vi "ReadEncDrive.vi"(5 "Teleop Local Data":T1 {"Vision"."Theta_Y" format="%.1f"; "Vision"."Theta_X" format="%.1f"; "Potentio" format="%.1f"; "Drive_Enc_R" format="%.1f"; "Drive_Enc_L" format="%.1f"; "Gyro_Angle" format="%.1f"; "Encoder_Lift" format="%.1f"; "Motor_Lift" format="%.3f"; "Motor_Intake" format="%.3f"; "Drive_Twist" format="%.3f"; "Drive_Forward" format="%.3f"}, 9 "error in":errorcluster) -> (6 "Teleop Local Data Out":T1 {"Vision"."Theta_Y" format="%.1f"; "Vision"."Theta_X" format="%.1f"; "Potentio" format="%.1f"; "Drive_Enc_R" format="%.1f"; "Drive_Enc_L" format="%.1f"; "Gyro_Angle" format="%.1f"; "Encoder_Lift" format="%.1f"; "Motor_Lift" format="%.3f"; "Motor_Intake" format="%.3f"; "Drive_Twist" format="%.3f"; "Drive_Forward" format="%.3f"}, 10 "error out":errorcluster)   [LabVIEW 2018]
uses:
  Typedefs/typedef_cluster_TeleOp_Local_Data.ctl
  Typedefs/typedef_cluster_Joystick.ctl
  Typedefs/typedef_cluster_Vision.ctl
  Typedefs/typedef_enum_refnums.ctl
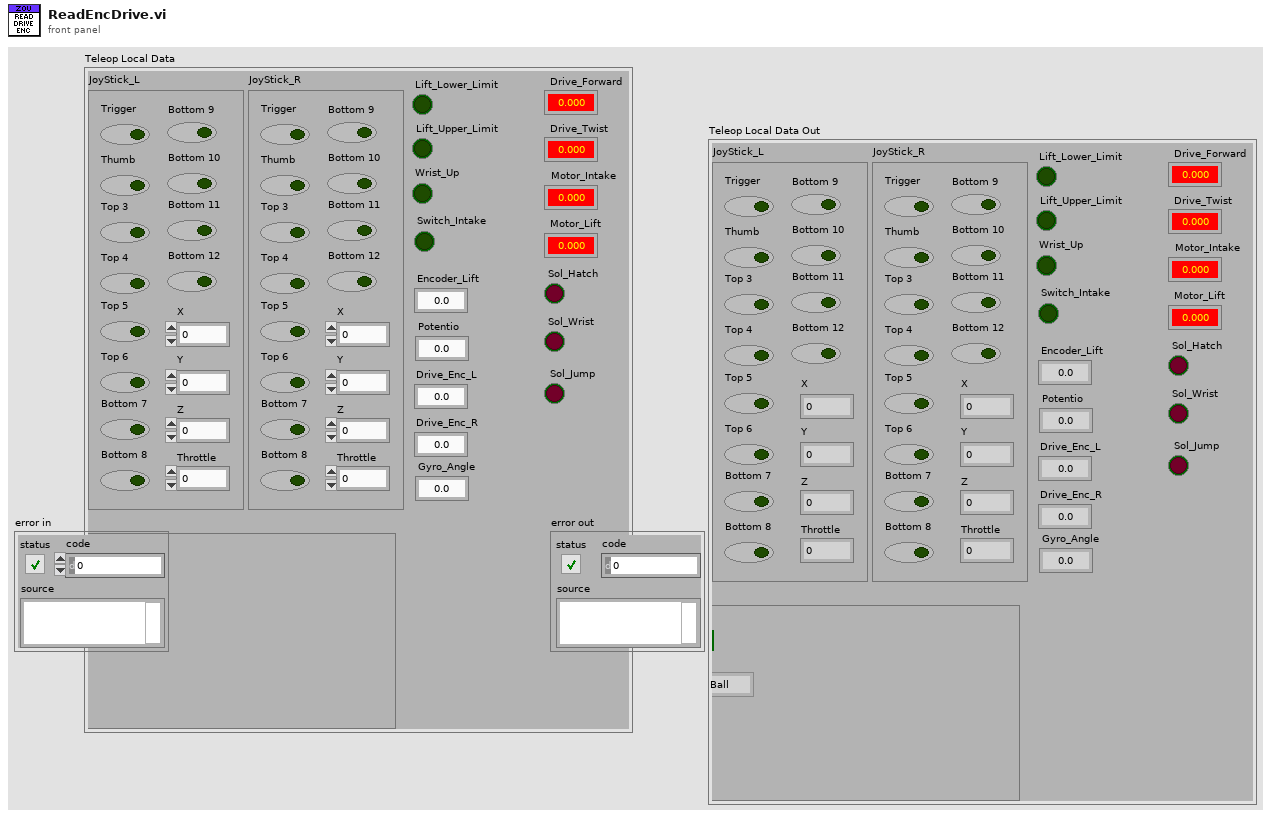
[diagram p1: front panel]
types:
  T1 = typedef "typedef_cluster_TeleOp_Local_Data.ctl" = cluster{"Lift_Lower_Limit":bool, "Wrist_Up":bool, "Switch_Intake":bool, "Encoder_Lift":dbl, "Sol_Wrist":bool, "Motor_Intake":dbl, "Motor_Lift":dbl, "Drive_Forward":dbl, "Drive_Twist":dbl, "Sol_Hatch":bool, "Gyro_Angle":dbl, "Drive_Enc_L":dbl, "Drive_Enc_R":dbl, "JoyStick_L":T2, "JoyStick_R":T2, "Potentio":dbl, "Vision":T3, "Lift_Upper_Limit":bool, "Sol_Jump":bool}
  T2 = typedef "typedef_cluster_Joystick.ctl" = cluster{"X":dbl, "Y":dbl, "Z":dbl, "Throttle":dbl, "Trigger":bool, "Thumb":bool, "Top 3":bool, "Top 4":bool, "Top 5":bool, "Top 6":bool, "Bottom 7":bool, "Bottom 8":bool, "Bottom 9":bool, "Bottom 10":bool, "Bottom 11":bool, "Bottom 12":bool}
  T3 = typedef "typedef_cluster_Vision.ctl" = cluster{"Theta_X":dbl, "Theta_Y":dbl, "Has_Target":bool, "Seek_Ball":bool, "Pipeline":enum16{"Ball", "Dual_Target", "Single_Target"}}
  T4 = typedef "typedef_enum_refnums.ctl" = enum16{"Joy_L", "Joy_R", "Drive_Motors", "Intake_Motor", "Wrist_Solenoid", "Hatch_Solenoid", "Compressor", "Lift_Motor", "Lift_Motor_2", "Gyro", "Drive_Enc_L", "Drive_Enc_R", "Lift_Lower_Limit", "Lift_Upper_Limit", "Ball_Switch", "Jump_Solenoid"}
  T5 = typedef "WPI_EncoderDevRef.ctl" = cluster{"DevStatus":errorcluster, "EncoderIndex":T6, "CounterIndex":T7, "DistancePerCount":dbl, "Decoding Type":T8}
  T6 = typedef "FPGA_EncoderIdx.ctl" = enum8{"Enc 0", "Enc 1", "Enc 2", "Enc 3", "Enc 4", "Enc 5", "Enc 6", "Enc 7", "Invalid"}
  T7 = typedef "FPGA_CounterCtrSystemIndex.ctl" = enum8{"Ctr 0", "Ctr 1", "Ctr 2", "Ctr 3", "Ctr 4", "Ctr 5", "Ctr 6", "Ctr 7", "Invalid"}
  T8 = typedef "WPI_EncoderType.ctl" = enum16{"1x", "2x", "4x"}
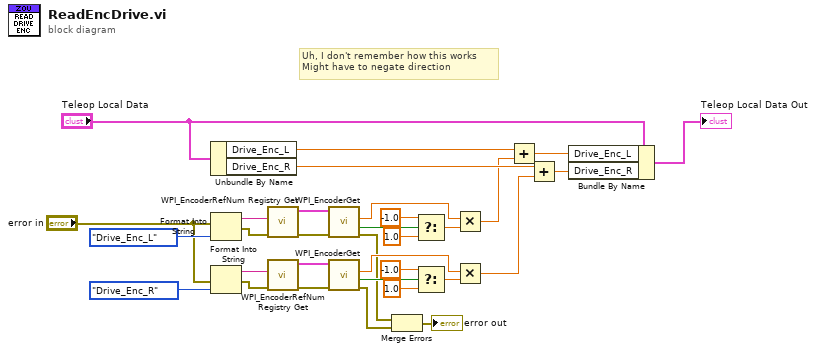
[diagram p0: block diagram]
diagram:
  # "Uh, I don't remember how this works\nMight have to negate direction"
  n1 = Unbundle By Name("Teleop Local Data") -> ("Drive_Enc_L"=w11:dbl, "Drive_Enc_R"=w12:dbl)
  n2 = Format Into String(error in="error in", typedef_enum_refnums."Drive_Enc_L" ("Enum")) -> (resulting string=w30:string, error out=w7:errorcluster)  [unwired: 2 in]
  n3 = Format Into String(error in="error in", typedef_enum_refnums."Drive_Enc_R" ("Enum")) -> (resulting string=w29:string, error out=w5:errorcluster)  [unwired: 2 in]
  n4 = call <vilib>:"WPI_EncoderRefNum Registry Get.vi"("error in (no error)"=w7, "refnum name"=w30) -> ("error out"=w6:errorcluster, "EncoderDevRef"=w27:T5)  [unwired: 8 in]
  n5 = call <vilib>:"WPI_EncoderRefNum Registry Get.vi"("error in (no error)"=w5, "refnum name"=w29) -> ("error out"=w4:errorcluster, "EncoderDevRef"=w28:T5)  [unwired: 8 in]
  n6 = call <vilib>:"WPI_EncoderGet.vi"("error in (no error)"=w6, "EncoderDevRef"=w27) -> ("error out"=w3:errorcluster, "Direction"=w22:bool, "Distance"=w20:dbl)  [unwired: 4 in, 3 out]
  n7 = call <vilib>:"WPI_EncoderGet.vi"("error in (no error)"=w4, "EncoderDevRef"=w28) -> ("error out"=w2:errorcluster, "Direction"=w16:bool, "Distance"=w15:dbl)  [unwired: 4 in, 3 out]
  n8 = Merge Errors(w3, w2) -> (→"error out":errorcluster)
  n9 = Select(t=-1.0, s=w22, f=1.0) -> (s? t:f=w21:dbl)
  n10 = Select(t=-1.0, s=w16, f=1.0) -> (s? t:f=w19:dbl)
  n11 = Multiply(x=w20, y=w21) -> (x*y=w10:dbl)
  n12 = Multiply(x=w15, y=w19) -> (x*y=w9:dbl)
  n13 = Add(x=w11, y=w10) -> (x+y=w14:dbl)
  n14 = Add(x=w12, y=w9) -> (x+y=w13:dbl)
  n15 = Bundle By Name(cluster="Teleop Local Data", "Drive_Enc_L"=w14, "Drive_Enc_R"=w13) -> (→"Teleop Local Data Out":T1)
